vi "GetChildren__slk_tc.vi"(0 "tree control in":refnum<class "TreeControl.lvclass">, 5 "parent tag (\"\")":string, 11 "error in (no error)":errorcluster, 12 "use current (T)":bool=TRUE) -> (4 "tree control out":refnum<class "TreeControl.lvclass">, 6 "children tags":string[](array[string]), 15 "error out":errorcluster)   [LabVIEW 2020, in "TreeControl.lvclass"]
doc: "Collects and returns all tags of parents immediate children. If the parent tag is an empty string, the currently selected item is used."
uses:
  Library/TreeControl.lvclass
  Library/TreeControl.lvclass/TreeControl.ctl
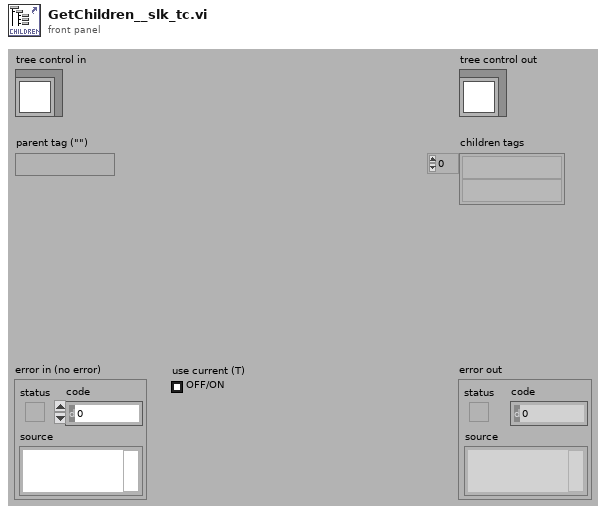
[diagram p1: front panel]
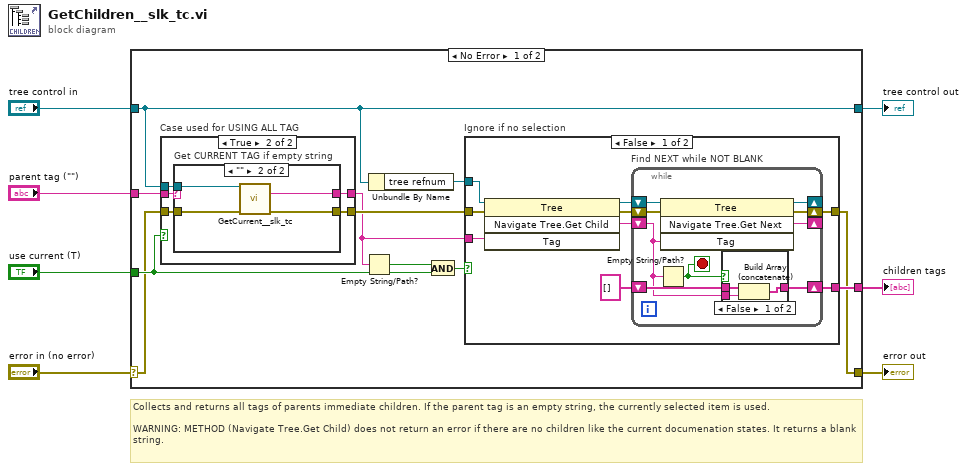
[diagram p0: block diagram]
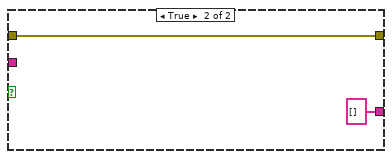
[diagram p3: hidden frame]
diagram:
  # "Collects and returns all tags of parents immediate children. If the parent tag is an empty string, the currently selected item is used. \n\nWARNING: METHOD (Navigate Tree.Get Child) does not return an error if there are no children like the current documenation states. It returns a blank string."
  n1 = case shown="No Error" "error in (no error)" {
    selector: "error in (no error)" -> [w9 w57]
    tunnel: [w8 w57] -> w6
    tunnel: [w14 w56] -> w4
    tunnel: "tree control in" -> [w14 w56]
    tunnel: "use current (T)" -> [w16 _]
    tunnel: "parent tag (\"\")" -> [w18 _]
    tunnel: [w10 _] -> w1
    frame No Error {
      n2 = case "Case used for USING ALL TAG" shown="True" w16 {
        tunnel: w18 -> [w44 w49]
        tunnel: w14 -> [_ w48]
        tunnel: w9 -> [w43 w47]
        tunnel: [w43 w46] -> w13
        tunnel: [w44 w45] -> w11
        frame False {
        }
        frame True {
          n3 = case "Get CURRENT TAG if empty string" shown="\"\"" w49 {
            selector: w49 -> [w51 _]
            tunnel: [w51 w55] -> w45
            tunnel: w48 -> [_ w54]
            tunnel: w47 -> [w50 w53]
            tunnel: [w50 w52] -> w46
            frame Default {
            }
            frame "" {
              n4 = call "GetCurrent__slk_tc.vi"("tree control in"=w54, "error in (no error)"=w53) -> ("current tag"=w55:string, "error out"=w52:errorcluster)  [unwired: 1 in, 11 out]
            }
          }
        }
      }
      n5 = Empty String/Path?(string/path=w11) -> (empty?=w17:bool)
      n6 = Unbundle By Name(w14) -> ("tree refnum"=w12:refnum<vi>)
      n7 = And(x=w17, y=w16) -> (x .and. y?=w15:bool)
      n8 = case "Ignore if no selection" shown="False" w15 {
        tunnel: w13 -> [w27 w42]
        tunnel: w12 -> [w26 _]
        tunnel: w11 -> [w25 _]
        tunnel: [w20 w42] -> w8
        tunnel: [w19 string[] []] -> w10
        frame False {
          n9 = invoke class="Tree" method="Navigate Tree.Get Child"(reference=w26, error in=w27, "Tag"=w25) -> (reference out=w23:refnum<vi>, error out=w24:errorcluster, "Navigate Tree:Get Child"=w22:string)  [unwired: 1 in, 1 out]
          n10 = while "Find NEXT while NOT BLANK" {
            shift-right: [w33] -> w20
            shift-left: w24 -> [w35]
            shift-right: [w34] -> _
            shift-left: w23 -> [w36]
            shift-right: [w32] -> _
            shift-left: w22 -> [w29]
            shift-right: [w30] -> w19
            shift-left: string[] [] -> [w31]
            stop <- w28 stop-if-true
            n11 = Empty String/Path?(string/path=w29) -> (empty?=w28:bool)
            n12 = invoke class="Tree" method="Navigate Tree.Get Next"(reference=w36, error in=w35, "Tag"=w29) -> (reference out=w34:refnum<vi>, error out=w33:errorcluster, "Navigate Tree:Get Next Item"=w32:string)  [unwired: 1 in, 1 out]
            n13 = case shown="False" w28 {
              tunnel: w31 -> [w39 w40]
              tunnel: [w38 w40] -> w30
              tunnel: w29 -> [w37 _]
              frame False {
                n14 = Build Array (concatenate)(w39, w37) -> (w38:string[])
              }
              frame True {
              }
            }
          }
        }
        frame True {
        }
      }
    }
    frame Error {
    }
  }
  "error out" <- w6
  "tree control out" <- w4
  "children tags" <- w1
